vi "Decorate And Unified Msgs.vi"(9 "Persistent Layers":refnum<class "Actor.lvclass">[](array[class]), 10 "Local Layers":refnum<class "Actor.lvclass">[](array[class])) -> (1 "Unified Msgs":T1, 2 "Unified Actor":refnum<class "Actor.lvclass">)   [LabVIEW 2025, in "jettl.lvlib"]
uses:
  jettl.lvlib
  Actor/Actor.lvclass
  Msgs.ctl
  Msg/Msg.lvclass
  Base Actor/Base Actor.lvlib
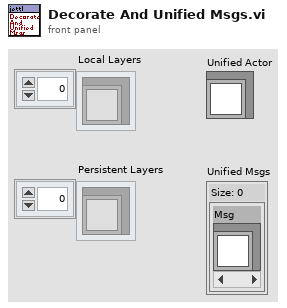
[diagram p1: front panel]
types:
  T1 = typedef "jettl.lvlib/Msgs.ctl" = set{refnum<class "Msg.lvclass">}
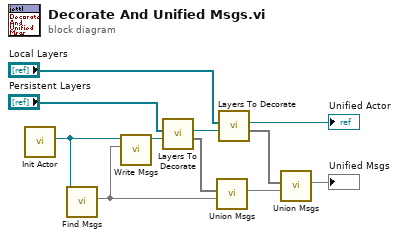
[diagram p0: block diagram]
diagram:
  n1 = call "Init Actor.vi"() -> ("Actor"=w7:refnum<class "Actor.lvclass">)  [unwired: 11 in]
  n2 = call-dynamic "Find Msgs.vi"("Actor in"=w7) -> ("Msgs"=w4:T1)  [unwired: 10 in]
  n3 = call-dynamic "Write Msgs.vi"("Msgs"=w4, "Actor in"=w7) -> ("Actor out"=w6:refnum<class "Actor.lvclass">)  [unwired: 9 in]
  n4 = call "Layers To Decorate.vi"("Actor To Decorate"=w6, "Layers"="Persistent Layers") -> ("Msgs"=w5:T1[], "Decorated Actor"=w11:refnum<class "Actor.lvclass">)  [unwired: 8 in]
  n5 = call "Union Msgs.vi"(9:"Msgs"=w4, 10:"Msgs"=w5) -> ("Union of Msgs"=w3:T1)  [unwired: 9 in]
  n6 = call "Layers To Decorate.vi"("Actor To Decorate"=w11, "Layers"="Local Layers") -> ("Msgs"=w2:T1[], "Decorated Actor"=→"Unified Actor":refnum<class "Actor.lvclass">)  [unwired: 8 in]
  n7 = call "Union Msgs.vi"(9:"Msgs"=w3, 10:"Msgs"=w2) -> ("Union of Msgs"=→"Unified Msgs":T1)  [unwired: 9 in]
